vi "Step ADD IR W Parameters.vi"(0 "VISA resource name":refnum<visa-resource-name>, 1 "Scanner Settings":T2={"Scan1"=1, "Scan2"=1, "Scan3"=1, "Scan4"=1, "Scan5"=1, "Scan6"=1, "Scan7"=1, "Scan8"=1, "Scan9"=1, "Scan10"=1, "Scan11"=1, "Scan12"=1, "Scan13"=1, "Scan14"=1, "Scan15"=1, "Scan16"=1} {"Scan16" scale=0.0..2.0; "Scan15" scale=0.0..2.0; "Scan14" scale=0.0..2.0; "Scan13" scale=0.0..2.0; "Scan12" scale=0.0..2.0; "Scan11" scale=0.0..2.0; "Scan10" scale=0.0..2.0; "Scan9" scale=0.0..2.0; "Scan8" scale=0.0..2.0; "Scan7" scale=0.0..2.0; "Scan6" scale=0.0..2.0; "Scan5" scale=0.0..2.0; "Scan4" scale=0.0..2.0; "Scan3" min=0 max=2 scale=0.0..2.0; "Scan2" min=0 max=2 scale=0.0..2.0; "Scan1" min=0 max=2 scale=0.0..2.0}, 2 "Internal scanner?":bool, 5 "IR Test Parameters In":T1={"Voltage (10~3000V)"=500, "High Limit(0.0, 0.1~50,000 Mohms)"=0.0, "Low Limit(0.1~50,000 Mohms)"=10.0, "Ramp Up Time (0.1~999.9 seconds)"=0.1, "Delay Time (0.5~999.9 seconds)"=0.5, "Ramp Down Time (0.0, 1.0~999.9 seconds)"=0.0, "Charge LO  (0.000~3.500uA)"=0.0, "Auto Charge LO (F: Off)"=FALSE, "Dwell Time (0.5~999.9 seconds, 0 = Constant)"=0.5} {"Dwell Time (0.5~999.9 seconds, 0 = Constant)" format="%.1f"; "Ramp Down Time (0.0, 1.0~999.9 seconds)" format="%.1f"; "Charge LO  (0.000~3.500uA)" format="%.2f"; "Delay Time (0.5~999.9 seconds)" format="%.1f"; "Ramp Up Time (0.1~999.9 seconds)" format="%.1f"; "Low Limit(0.1~50,000 Mohms)" format="%.1f"; "High Limit(0.0, 0.1~50,000 Mohms)" format="%.1f"}, 7 "Step Selection (1-200)":i32=1, 9 "Add Step":bool, 11 "error in (no error)":errorcluster) -> (4 "VISA resource name out":refnum<visa-resource-name>, 15 "error out":errorcluster)   [LabVIEW 2020, in "eec EST 300.lvlib"]
doc: "Inserts a IR test with the User defined parameters into the assigned Step Selecton.\n\nIf Add step is set to Edit, it will replace the existing step. If it is set to Add it will insert the new step and increment all steps after the selected step by 1.\n\nSee specifications for Limits."
uses:
  <instrlib>/eec EST 300/eec EST 300.lvlib
  <instrlib>/eec EST 300/Public/Configure/Steps/Low Level/Scanner Settings.ctl
  <instrlib>/eec EST 300/Public/Configure/Steps/Low Level/IR Test Parameters.ctl
panel:
  # "Add"
  # "Edit"
  # "On\nOff"
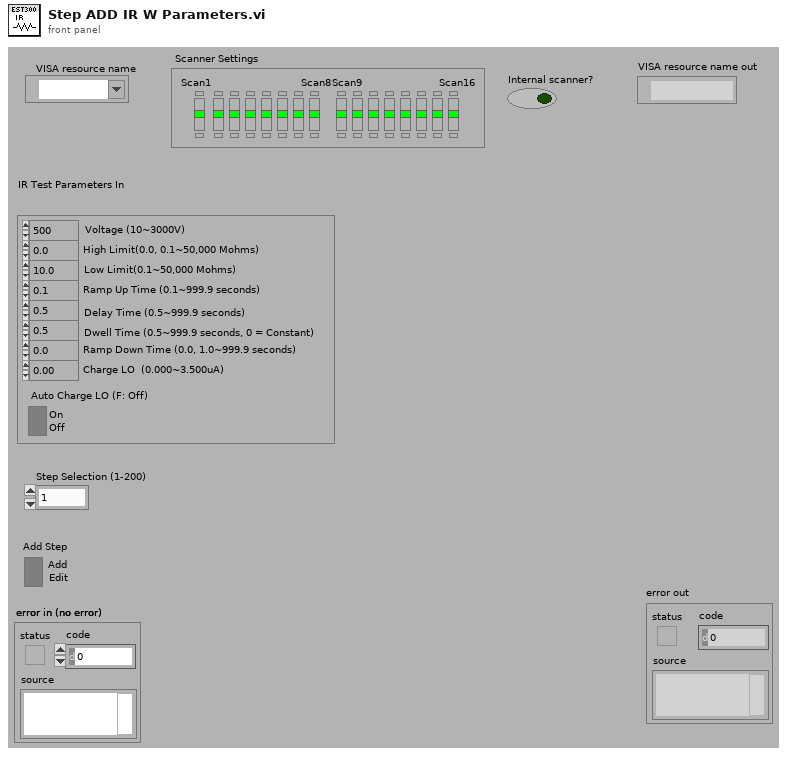
[diagram p1: front panel]
types:
  T1 = typedef "eec EST 300.lvlib/IR Test Parameters.ctl" = cluster{"Voltage (10~3000V)":i64, "High Limit(0.0, 0.1~50,000 Mohms)":dbl, "Low Limit(0.1~50,000 Mohms)":dbl, "Ramp Up Time (0.1~999.9 seconds)":dbl, "Delay Time (0.5~999.9 seconds)":dbl, "Ramp Down Time (0.0, 1.0~999.9 seconds)":dbl, "Charge LO  (0.000~3.500uA)":dbl, "Auto Charge LO (F: Off)":bool, "Dwell Time (0.5~999.9 seconds, 0 = Constant)":dbl}
  T2 = typedef "eec EST 300.lvlib/Scanner Settings.ctl" = cluster{"Scan1":i32, "Scan2":i32, "Scan3":i32, "Scan4":i32, "Scan5":i32, "Scan6":i32, "Scan7":i32, "Scan8":i32, "Scan9":i32, "Scan10":i32, "Scan11":i32, "Scan12":i32, "Scan13":i32, "Scan14":i32, "Scan15":i32, "Scan16":i32}
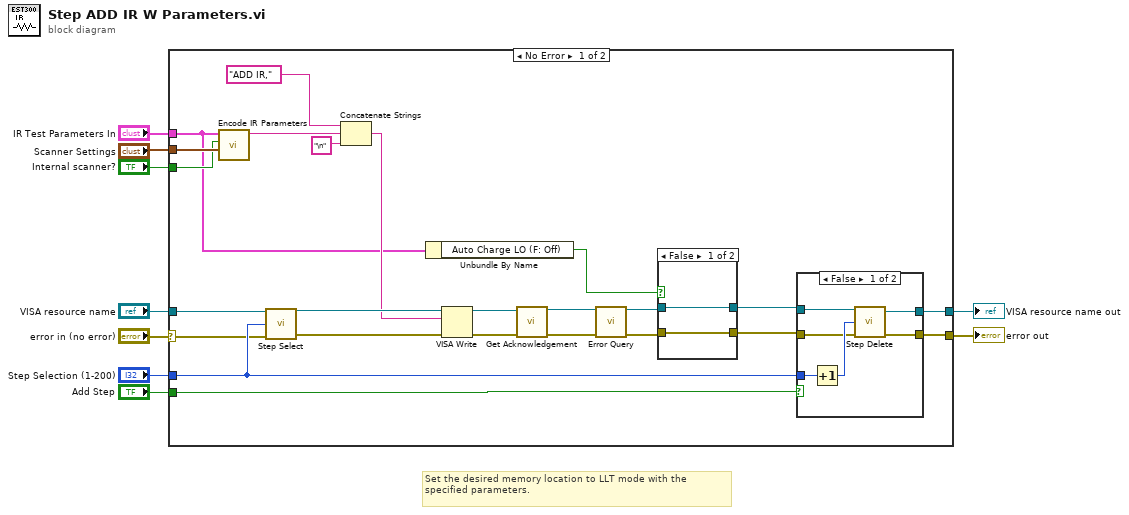
[diagram p0: block diagram]
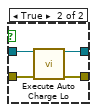
[diagram p2: hidden frame]
diagram:
  # "Set the desired memory location to LLT mode with the specified parameters."
  n1 = case shown="No Error" "error in (no error)" {
    selector: "error in (no error)" -> [w22 w49]
    tunnel: [w31 w49] -> w8
    tunnel: [w30 w48] -> w6
    tunnel: "VISA resource name" -> [w23 w48]
    tunnel: "Step Selection (1-200)" -> [w24 _]
    tunnel: "Add Step" -> [w29 _]
    tunnel: "Scanner Settings" -> [w14 _]
    tunnel: "Internal scanner?" -> [w13 _]
    tunnel: "IR Test Parameters In" -> [w11 _]
    frame No Error {
      n2 = call <instrlib>:"Encode IR Parameters.vi"("Scanner Settings In"=w14, "Internal Scanner Exists?"=w13, "IR Test Parameters In"=w11) -> ("ADD command"=w12:string)  [unwired: 6 in, 2 out]
      n3 = call <instrlib>:"Step Select.vi"("VISA resource name"=w23, "Step Number (1)"=w24, "error in (no error)"=w22) -> ("VISA resource name out"=w32:refnum<visa-resource-name>, "error out"=w33:errorcluster)  [unwired: 11 in]
      n4 = Concatenate Strings("ADD IR," ("string"), w12, "\n" ("string")) -> (w27:string)
      n5 = Unbundle By Name(w11) -> ("Auto Charge LO (F: Off)"=w10:bool)
      n6 = VISA Write(VISA resource name=w32, write buffer=w27, error in (no error)=w33) -> (VISA resource name out=w20:refnum<visa-resource-name>, error out=w19:errorcluster)  [unwired: 1 out]
      n7 = call <instrlib>:"Get Acknowledgement.vi"("VISA resource name"=w20, "error in (no error)"=w19) -> ("VISA resource name out"=w26:refnum<visa-resource-name>, "error out"=w25:errorcluster)  [unwired: 12 in]
      n8 = call <instrlib>:"Error Query.vi"("VISA resource name"=w26, "error in (no error)"=w25) -> ("VISA resource name out"=w18:refnum<visa-resource-name>, "error out"=w17:errorcluster)  [unwired: 10 in, 2 out]
      n9 = case shown="False" w10 {
        tunnel: w18 -> [w35 w39]
        tunnel: w17 -> [w34 w38]
        tunnel: [w35 w37] -> w15
        tunnel: [w34 w36] -> w16
        frame False {
        }
        frame True {
          n10 = call <instrlib>:"Execute Auto Charge Lo.vi"("VISA resource name"=w39, "error in (no error)"=w38) -> ("VISA resource name out"=w37:refnum<visa-resource-name>, "error out"=w36:errorcluster)  [unwired: 12 in]
        }
      }
      n11 = case shown="False" w29 {
        tunnel: w24 -> [w45 _]
        tunnel: w16 -> [w43 w46]
        tunnel: w15 -> [w42 w47]
        tunnel: [w41 w46] -> w31
        tunnel: [w40 w47] -> w30
        frame False {
          n12 = Increment(x=w45) -> (x+1=w44:i32)
          n13 = call <instrlib>:"Step Delete.vi"("VISA resource name"=w42, "Step Number (0 = Active Step)"=w44, "error in (no error)"=w43) -> ("VISA resource name out"=w40:refnum<visa-resource-name>, "error out"=w41:errorcluster)  [unwired: 11 in]
        }
        frame True {
        }
      }
    }
    frame Error {
    }
  }
  "error out" <- w8
  "VISA resource name out" <- w6
